vi "Read Movie Appearances.vi"(8 "error in (no error)":errorcluster, 11 "Chevy Chase in":refnum<class "Chevy Chase.lvclass">) -> (0 "error out":errorcluster, 2 "Movie Appearances":string, 3 "Chevy Chase out":refnum<class "Chevy Chase.lvclass">)   [LabVIEW 2019, in "Chevy Chase.lvclass"]
uses:
  Chevy Chase.lvclass
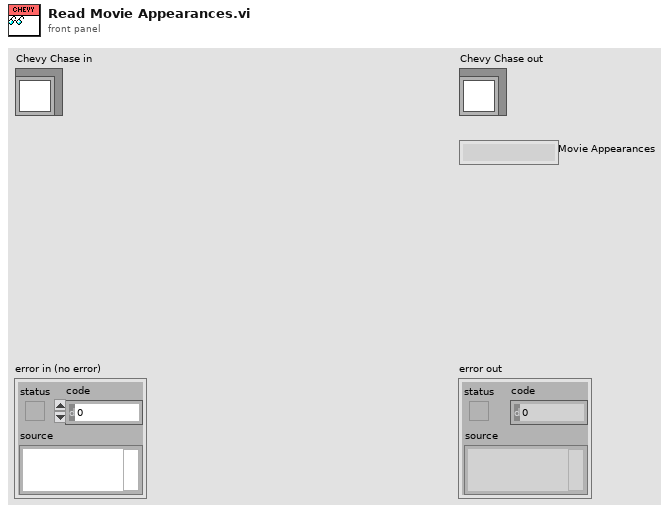
[diagram p1: front panel]
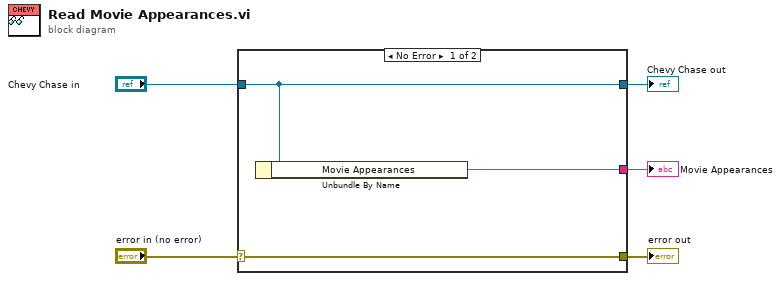
[diagram p0: block diagram]
diagram:
  n1 = case shown="No Error" "error in (no error)" {
    selector: "error in (no error)" -> [w8 w9]
    tunnel: [w8 w9] -> w4
    tunnel: [w7 w10] -> w2
    tunnel: "Chevy Chase in" -> [w7 w10]
    tunnel: [w6 _] -> w1
    frame No Error {
      n2 = Unbundle By Name(w7) -> ("Movie Appearances"=w6:string)
    }
    frame Error {
    }
  }
  "error out" <- w4
  "Chevy Chase out" <- w2
  "Movie Appearances" <- w1
